vi "myPICO_Run.vi"(6 "实际驱动台数":u16, 7 "stop":bool, 8 "簇 3":T2, 9 "簇 4":T2, 10 "n_tbase":u32, 11 "n_samp":u64) -> (0 "MultiBuffers (Max or non-aggregated) 2":T1(array[cluster]), 1 "MultiBuffers (Max or non-aggregated)":T1(array[cluster]), 2 "簇 2":T4, 3 "簇":T4, 5 "布尔输出":bool)   [LabVIEW 2024]
uses:
  shared/PicoBuffers.ctl
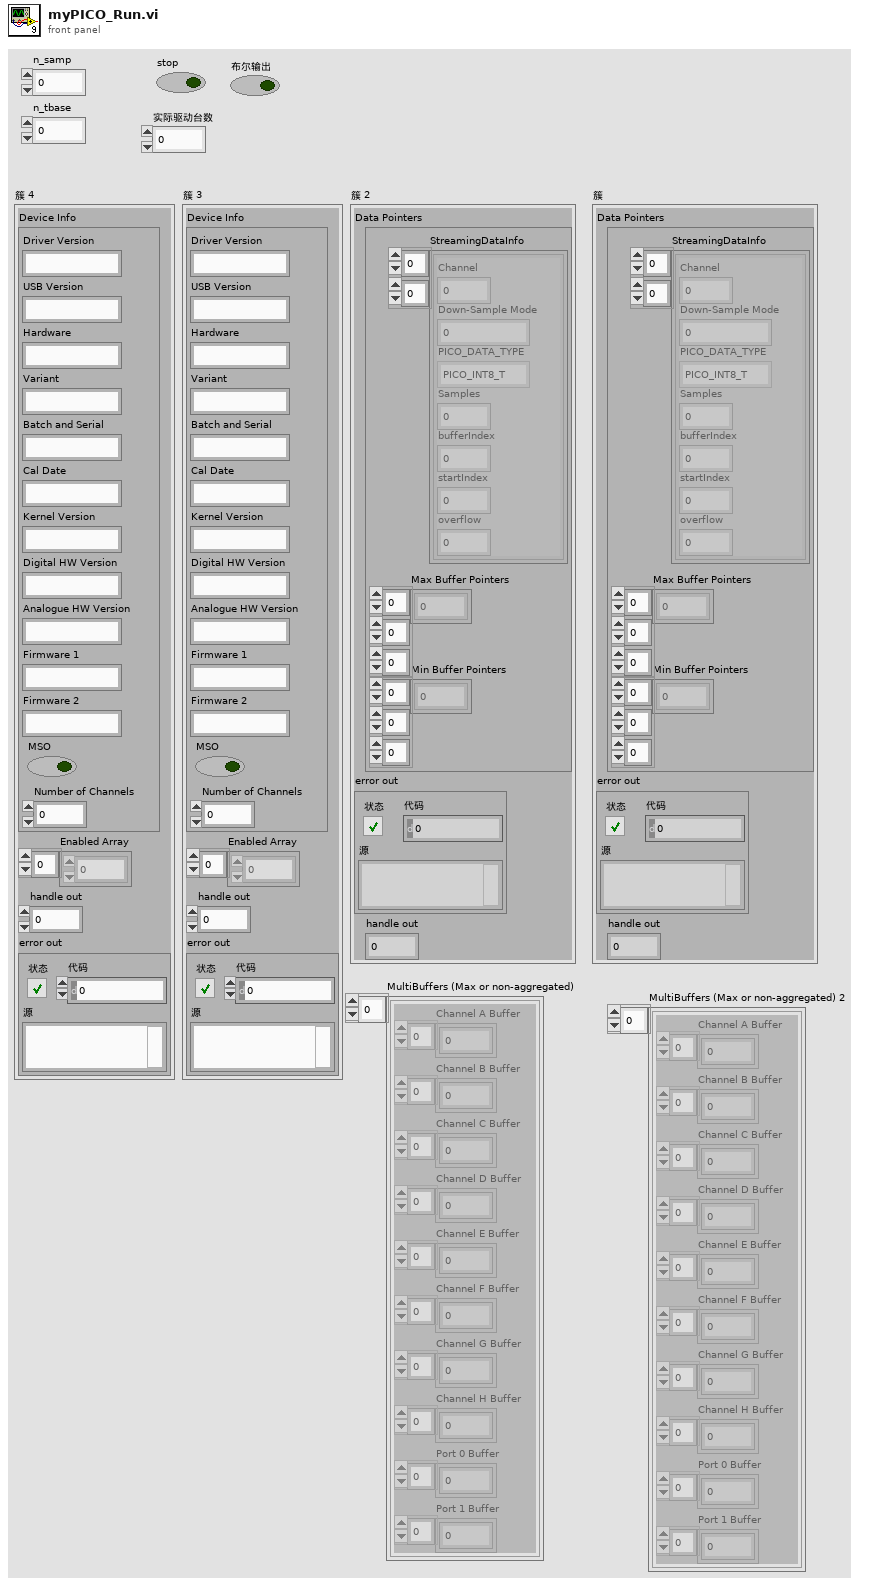
[diagram p1: front panel]
types:
  T1 = cluster{"Channel A Buffer":i16[], "Channel B Buffer":i16[], "Channel C Buffer":i16[], "Channel D Buffer":i16[], "Channel E Buffer":i16[], "Channel F Buffer":i16[], "Channel G Buffer":i16[], "Channel H Buffer":i16[], "Port 0 Buffer":i16[], "Port 1 Buffer":i16[]}[]
  T2 = cluster{"Device Info":cluster{"Driver Version":string, "USB Version":string, "Hardware":string, "Variant":string, "Batch and Serial":string, "Cal Date":string, "Kernel Version":string, "Digital HW Version":string, "Analogue HW Version":string, "Firmware 1":string, "Firmware 2":string, "MSO":bool, "Number of Channels":i16}, "Enabled Array":i16[], "handle out":i16, "error out":errorcluster}
  T3 = typedef "PicoBuffers.ctl" = cluster{"Max Buffer Pointers":u64[][][], "Min Buffer Pointers":u64[][][], "StreamingDataInfo":cluster{"Channel":u32, "Down-Sample Mode":u32, "PICO_DATA_TYPE":enum32{"PICO_INT8_T", "PICO_INT16_T", "PICO_INT32_T", "PICO_UINT32_T", "PICO_INT64_T", ""}, "Samples":i32, "bufferIndex":u64, "startIndex":i32, "overflow":i16}[][]}
  T4 = cluster{"Data Pointers":T3, "error out":errorcluster, "handle out":i16}
  T5 = cluster{"Driver Version":string, "USB Version":string, "Hardware":string, "Variant":string, "Batch and Serial":string, "Cal Date":string, "Kernel Version":string, "Digital HW Version":string, "Analogue HW Version":string, "Firmware 1":string, "Firmware 2":string, "MSO":bool, "Number of Channels":i16}
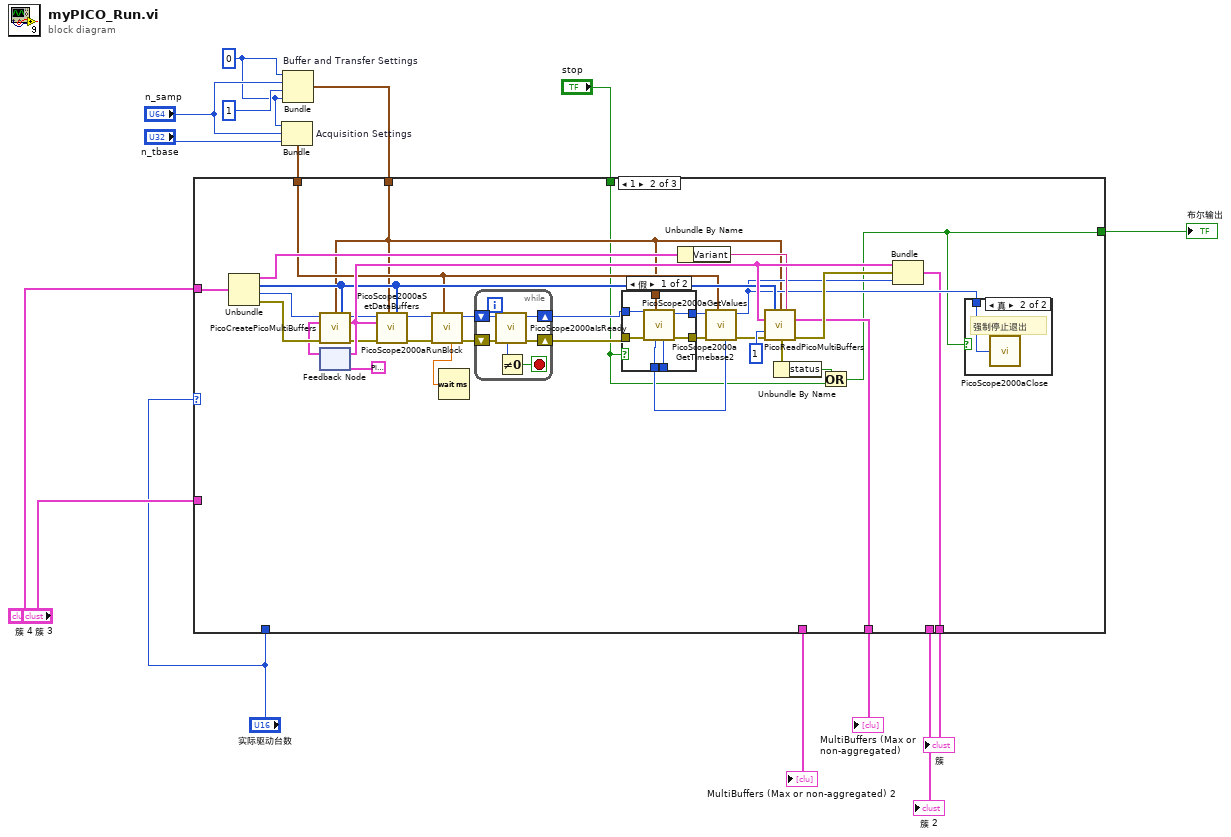
[diagram p0: block diagram]
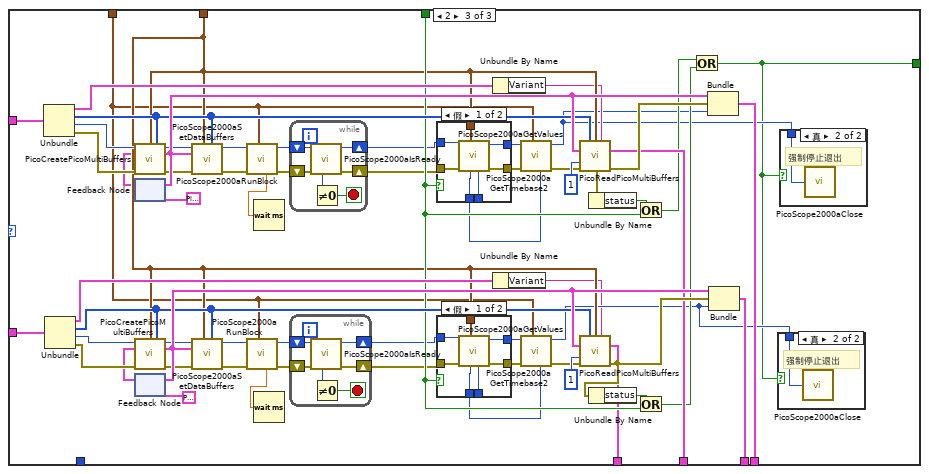
[diagram p5: hidden frame]
diagram:
  w3 = u64 0
  n1 = Bundle "Acquisition Settings"(w3, "n_samp"="n_samp", "n_tbase"="n_tbase") -> (w5:cluster{u64, "n_samp":u64, "n_tbase":u32})  [unwired: 1 in]
  n2 = Bundle "Buffer and Transfer Settings"(w3, "n_samp"="n_samp", u64 1, w3) -> (w6:cluster{u64, "n_samp":u64, u64, u64})  [unwired: 1 in]
  n3 = case shown="1" "实际驱动台数" {
    tunnel: [_ w18 w122] -> w15
    tunnel: [_ _ w121] -> w14
    tunnel: "簇 3" -> [_ _ w113]
    tunnel: "簇 4" -> [_ w21 w108]
    tunnel: "stop" -> [w16 w20 w107]
    tunnel: [_ w19 w106] -> w10
    tunnel: [_ _ w105] -> w9
    tunnel: w6 -> [_ w22 w102]
    tunnel: w5 -> [_ w23 w101]
    tunnel: "实际驱动台数" -> [_ _ _]
    tunnel: [w16 w17 w81] -> w2
    frame 0, Default {
    }
    frame 1 {
      n4 = Unbundle(w21) -> ("Device Info"=w45:T5, "Enabled Array"=w44:i16[], "handle out"=w43:i16, "error out"=w42:errorcluster)
      n5 = feedback #1(T3 {"Max Buffer Pointers"=[], "Min Buffer Pointers"=[], "StreamingDataInfo"=[]} ("Data Pointers")) -> (w40:T3)
      n6 = call "PicoCreatePicoMultiBuffers.vi"("Buffer and Transfer Settings"=w22, "enabled array"=w44, "Data Pointers In"=w40, "error in (no error)"=w42) -> ("Data Pointers"=w46:T3, "error out"=w39:errorcluster)  [unwired: 10 in]
      n7 = feedback-in #1(w46) -> ()
      n8 = call "PicoScope2000aSetDataBuffers.vi"("enabled array"=w44, "Buffer and Transfer Settings"=w22, "error in (no error)"=w39, "Data Pointers In"=w46, "handle in"=w43) -> ("error out"=w37:errorcluster, "handle out"=w38:i16)  [unwired: 5 in]
      n9 = call "PicoScope2000aRunBlock.vi"("Acquisition Settings"=w23, "error in (no error)"=w37, "handle in"=w38) -> ("error out"=w26:errorcluster, "handle out"=w27:i16, "timeIndisposedMs"=w32:dbl)  [unwired: 5 in, 1 out]
      n10 = Wait (ms)(milliseconds to wait=w32) -> ()  [unwired: 1 out]
      n11 = while {
        shift-right: [w62] -> w30
        shift-left: w26 -> [w63]
        shift-right: [w61] -> w29
        shift-left: w27 -> [w60]
        stop <- w58 stop-if-true
        n12 = call "PicoScope2000aIsReady.vi"("error in (no error)"=w63, "handle in"=w60) -> ("error out"=w62:errorcluster, "handle out"=w61:i16, "ready"=w59:i16)  [unwired: 7 in]
        n13 = Not Equal To 0?(x=w59) -> (x != 0?=w58:bool)
      }
      n14 = case shown="假" w20 {
        tunnel: w30 -> [w55 w56]
        tunnel: w29 -> [w54 w57]
        tunnel: [w53 w57] -> w34
        tunnel: [w52 w56] -> w33
        tunnel: w22 -> [w51 _]
        tunnel: [w50 _] -> _
        tunnel: [w49 _] -> w31
        frame False {
          n15 = call "PicoScope2000aGetValues.vi"("Buffer and Transfer Settings"=w51, "error in (no error)"=w55, "handle in"=w54) -> ("error out"=w52:errorcluster, "handle out"=w53:i16, "overflow"=w50:i16, "noOfSamples"=w49:u64)  [unwired: 5 in]
        }
        frame True {
        }
      }
      n16 = Unbundle By Name(w45) -> ("Variant"=w28:string)
      n17 = call "PicoScope2000aGetTimebase2.vi"("Number of Samples"=w31, "Acquisition Settings"=w23, "error in (no error)"=w33, "handle in"=w34) -> ("error out"=w35:errorcluster, "handle out"=w24:i16)  [unwired: 5 in, 1 out]
      n18 = call "PicoReadPicoMultiBuffers.vi"("enabled array"=w44, "Buffer and Transfer Settings"=w22, "Variant"=w28, "Data Pointers"=w46, "No of Buffers"=1, "error in (no error)"=w35) -> ("MultiBuffers (Max or non-aggregated)"=w19:T1, "error out"=w47:errorcluster)  [unwired: 7 in, 1 out]
      n19 = Unbundle By Name(w47) -> ("status"=w25:bool)
      n20 = Or(x=w25, y=w20) -> (x .or. y?=w17:bool)
      n21 = Bundle("Data Pointers"=w46, "error out"=w47, "handle out"=w24) -> (w18:T4)  [unwired: 1 in]
      n22 = case shown="真" w17 {
        tunnel: w24 -> [_ w48]
        frame False {
        }
        frame True {
          # "强制停止退出"
          n23 = call "PicoScope2000aClose.vi"("handle"=w48) -> ()
        }
      }
    }
    frame 2 {
      n24 = Unbundle(w108) -> ("Device Info"=w112:T5, "Enabled Array"=w111:i16[], "handle out"=w110:i16, "error out"=w109:errorcluster)
      n25 = Unbundle(w113) -> ("Device Info"=w117:T5, "Enabled Array"=w116:i16[], "handle out"=w115:i16, "error out"=w114:errorcluster)
      n26 = feedback #2(T3 {"Max Buffer Pointers"=[], "Min Buffer Pointers"=[], "StreamingDataInfo"=[]} ("Data Pointers")) -> (w99:T3)
      n27 = call "PicoCreatePicoMultiBuffers.vi"("Buffer and Transfer Settings"=w102, "enabled array"=w111, "Data Pointers In"=w99, "error in (no error)"=w109) -> ("Data Pointers"=w118:T3, "error out"=w98:errorcluster)  [unwired: 10 in]
      n28 = feedback-in #2(w118) -> ()
      n29 = feedback #3(T3 {"Max Buffer Pointers"=[], "Min Buffer Pointers"=[], "StreamingDataInfo"=[]} ("Data Pointers")) -> (w79:T3)
      n30 = call "PicoCreatePicoMultiBuffers.vi"("Buffer and Transfer Settings"=w102, "enabled array"=w116, "Data Pointers In"=w79, "error in (no error)"=w114) -> ("Data Pointers"=w119:T3, "error out"=w78:errorcluster)  [unwired: 10 in]
      n31 = feedback-in #3(w119) -> ()
      n32 = call "PicoScope2000aSetDataBuffers.vi"("enabled array"=w111, "Buffer and Transfer Settings"=w102, "error in (no error)"=w98, "Data Pointers In"=w118, "handle in"=w110) -> ("error out"=w96:errorcluster, "handle out"=w97:i16)  [unwired: 5 in]
      n33 = call "PicoScope2000aSetDataBuffers.vi"("enabled array"=w116, "Buffer and Transfer Settings"=w102, "error in (no error)"=w78, "Data Pointers In"=w119, "handle in"=w115) -> ("error out"=w76:errorcluster, "handle out"=w77:i16)  [unwired: 5 in]
      n34 = call "PicoScope2000aRunBlock.vi"("Acquisition Settings"=w101, "error in (no error)"=w96, "handle in"=w97) -> ("error out"=w85:errorcluster, "handle out"=w86:i16, "timeIndisposedMs"=w91:dbl)  [unwired: 5 in, 1 out]
      n35 = call "PicoScope2000aRunBlock.vi"("Acquisition Settings"=w101, "error in (no error)"=w76, "handle in"=w77) -> ("error out"=w65:errorcluster, "handle out"=w66:i16, "timeIndisposedMs"=w71:dbl)  [unwired: 5 in, 1 out]
      n36 = Wait (ms)(milliseconds to wait=w91) -> ()  [unwired: 1 out]
      n37 = Wait (ms)(milliseconds to wait=w71) -> ()  [unwired: 1 out]
      n38 = while {
        shift-right: [w154] -> w89
        shift-left: w85 -> [w155]
        shift-right: [w153] -> w88
        shift-left: w86 -> [w152]
        stop <- w150 stop-if-true
        n39 = call "PicoScope2000aIsReady.vi"("error in (no error)"=w155, "handle in"=w152) -> ("error out"=w154:errorcluster, "handle out"=w153:i16, "ready"=w151:i16)  [unwired: 7 in]
        n40 = Not Equal To 0?(x=w151) -> (x != 0?=w150:bool)
      }
      n41 = while {
        shift-right: [w137] -> w69
        shift-left: w65 -> [w138]
        shift-right: [w136] -> w68
        shift-left: w66 -> [w135]
        stop <- w133 stop-if-true
        n42 = call "PicoScope2000aIsReady.vi"("error in (no error)"=w138, "handle in"=w135) -> ("error out"=w137:errorcluster, "handle out"=w136:i16, "ready"=w134:i16)  [unwired: 7 in]
        n43 = Not Equal To 0?(x=w134) -> (x != 0?=w133:bool)
      }
      n44 = case shown="假" w107 {
        tunnel: w89 -> [w147 w148]
        tunnel: w88 -> [w146 w149]
        tunnel: [w145 w149] -> w93
        tunnel: [w144 w148] -> w92
        tunnel: w102 -> [w143 _]
        tunnel: [w142 _] -> _
        tunnel: [w141 _] -> w90
        frame False {
          n45 = call "PicoScope2000aGetValues.vi"("Buffer and Transfer Settings"=w143, "error in (no error)"=w147, "handle in"=w146) -> ("error out"=w144:errorcluster, "handle out"=w145:i16, "overflow"=w142:i16, "noOfSamples"=w141:u64)  [unwired: 5 in]
        }
        frame True {
        }
      }
      n46 = case shown="假" w107 {
        tunnel: w69 -> [w130 w131]
        tunnel: w68 -> [w129 w132]
        tunnel: [w128 w132] -> w73
        tunnel: [w127 w131] -> w72
        tunnel: w102 -> [w126 _]
        tunnel: [w125 _] -> _
        tunnel: [w124 _] -> w70
        frame False {
          n47 = call "PicoScope2000aGetValues.vi"("Buffer and Transfer Settings"=w126, "error in (no error)"=w130, "handle in"=w129) -> ("error out"=w127:errorcluster, "handle out"=w128:i16, "overflow"=w125:i16, "noOfSamples"=w124:u64)  [unwired: 5 in]
        }
        frame True {
        }
      }
      n48 = Unbundle By Name(w112) -> ("Variant"=w87:string)
      n49 = Unbundle By Name(w117) -> ("Variant"=w67:string)
      n50 = call "PicoScope2000aGetTimebase2.vi"("Number of Samples"=w90, "Acquisition Settings"=w101, "error in (no error)"=w92, "handle in"=w93) -> ("error out"=w94:errorcluster, "handle out"=w83:i16)  [unwired: 5 in, 1 out]
      n51 = call "PicoScope2000aGetTimebase2.vi"("Number of Samples"=w70, "Acquisition Settings"=w101, "error in (no error)"=w72, "handle in"=w73) -> ("error out"=w74:errorcluster, "handle out"=w82:i16)  [unwired: 5 in, 1 out]
      n52 = call "PicoReadPicoMultiBuffers.vi"("enabled array"=w111, "Buffer and Transfer Settings"=w102, "Variant"=w87, "Data Pointers"=w118, "No of Buffers"=1, "error in (no error)"=w94) -> ("MultiBuffers (Max or non-aggregated)"=w106:T1, "error out"=w123:errorcluster)  [unwired: 7 in, 1 out]
      n53 = call "PicoReadPicoMultiBuffers.vi"("enabled array"=w116, "Buffer and Transfer Settings"=w102, "Variant"=w67, "Data Pointers"=w119, "No of Buffers"=1, "error in (no error)"=w74) -> ("MultiBuffers (Max or non-aggregated)"=w105:T1, "error out"=w120:errorcluster)  [unwired: 7 in, 1 out]
      n54 = Unbundle By Name(w123) -> ("status"=w84:bool)
      n55 = Unbundle By Name(w120) -> ("status"=w64:bool)
      n56 = Or(x=w84, y=w107) -> (x .or. y?=w103:bool)
      n57 = Or(x=w64, y=w107) -> (x .or. y?=w104:bool)
      n58 = Or(x=w103, y=w104) -> (x .or. y?=w81:bool)
      n59 = Bundle("Data Pointers"=w118, "error out"=w123, "handle out"=w83) -> (w122:T4)  [unwired: 1 in]
      n60 = Bundle("Data Pointers"=w119, "error out"=w120, "handle out"=w82) -> (w121:T4)  [unwired: 1 in]
      n61 = case shown="真" w81 {
        tunnel: w82 -> [_ w139]
        frame False {
        }
        frame True {
          # "强制停止退出"
          n62 = call "PicoScope2000aClose.vi"("handle"=w139) -> ()
        }
      }
      n63 = case shown="真" w81 {
        tunnel: w83 -> [_ w140]
        frame False {
        }
        frame True {
          # "强制停止退出"
          n64 = call "PicoScope2000aClose.vi"("handle"=w140) -> ()
        }
      }
    }
  }
  "簇" <- w15
  "簇 2" <- w14
  "MultiBuffers (Max or non-aggregated)" <- w10
  "MultiBuffers (Max or non-aggregated) 2" <- w9
  "布尔输出" <- w2
